vi "Meas Process Record.vi"(5 "result string label":string="str res", 7 "session":T11={"adc"={"niScope"={"channel cfg"=[], "sessions"=[], "multi cards"=FALSE, "channels"=0, "type"=enum."n/a", "memory [B/chn]"=0, "ext. clock [Hz]"=0.0, "samples count"=0, "use streaming"=FALSE, "proc setup"={"packet size [smpl]"=0, "current timeout [s]"=0.0, "blk2blk timeout [s]"=0.0, "event time"=timestamp(0 s since 1904-01-01), "temp sampl T [s]"=0.0, "data queue"=refnum, "stop notifier"=refnum, "proc ref"=refnum}, "sample width [B]"=0, "ranges [V]"=[], "trigger setup"={"coupling"=1, "level [V]"=0.0, "slope"=0, "mode"=enum."Immediate", "pre-trigger [%]"=0.0}, "fs [Hz]"=0.0, "bitres [bit]"=0, "clock source"=enum."VAL_NO_SOURCE"}, "3458A"={"channels"=[], "sync unit"={"VISA"="", "type"=enum."Picotest U6200A"}, "awg unit"={"type"=enum."Agilent 331xxA to 332xxA", "VISA"="", "enable 10MHz ref"=FALSE, "cmi ckd2"={"VISA"="", "clock source"=enum."Auto", "manual ref clk"=FALSE, "ref clock [Hz]"=0.0, "div mode"=enum."Set divisor directly"}, "cmi sync v3"={"VISA"="", "baud rate [bd/s]"=115200, "source"=enum."Auto", "hv range"=enum."1kV", "fsrc is fixed"=FALSE, "fsrc [Hz]"=10000000.0, "freq integ [s]"=1.0, "freq filter"=5, "trig level"=enum."TTL 5V", "chn1 mode"=enum."Source divider", "chn1 level"=enum."Positive 5V", "chn2 mode"=enum."Source divider", "chn2 level"=enum."Positive 5V", "chn2 div"=1, "chn3 mode"=enum."Chn 1 Active", "chn3 level"=enum."Positive 5V", "chn1 div entry"=enum."Calculate nearest divisor from measured fx", "chn1 dev limit [%]"=1.0, "chn1 check dev"=FALSE}, "trigger"={"source"=enum."Immediate", "slope"=enum."POS", "coupling"=enum."DC", "level [V]"=0.0, "hysteresis [V]"=0.0, "pre-trigger [%]"=0.0}, "HMF2500 cfg"={"Baud Rate"=9600, "Parity"=0, "Data Bits"=8, "Flow Control"=4}}, "sync mode"=enum."MASTER-SLAVE, MASTER clocked by TIMER", "streaming mode"=FALSE, "idn mode"=enum."Auto", "sampling mode"=enum."DCV", "sample memory [B]"=0, "proc setup"={"channel id"=0, "packet size [smpl]"=0, "current timeout [s]"=0.0, "blk2blk timeout [s]"=0.0, "event time"=timestamp(0 s since 1904-01-01), "stop notifier"=refnum, "data queues"=[], "proc refs"=[], "bus semaphore"=refnum}, "sample size [B]"=0, "sample count"=0, "aux data"={"channel id"=0, "valid?"=[], "gain [V]"=[], "timestamp [s]"=[], "Ts [s]"=0.0, "abs timestamp"=timestamp(0 s since 1904-01-01), "t [deg C]"=[], "multiplex timestamp [s]"=-1.0, "only multiplex?"=FALSE, "multiplex smpl offset"=0, "overflow?"=FALSE}, "ranges [V]"=[], "aperture [s]"=0.0, "LEVEL trigger"={"edge"=enum."POS", "level [V]"=0.0, "coupling"=enum."DC"}, "trigger mode"=enum."AUTO", "measure temp.?"=FALSE, "disp mesages"=[], "shared bus?"=FALSE, "disable display?"=FALSE, "aper mode"=enum."Manual", "aper rules"=[], "multiplex"={"cycles"=0, "delay [s]"=0.0, "enabled"=FALSE, "overhead [s]"=1.0, "tot smpls"=0, "sub-rec"=0, "overhead [%]"=0.0, "emulated"=FALSE}, "F8588 lpf"=enum."Off", "F8588 pll"=enum."Off", "F8588 couple"=enum."DC, auto", "fs"={"freq mode"=enum."fs or Ts", "fs [Hz]"=0.0, "fref [Hz]"=0.0, "mul"=0.0, "div"=0.0}, "fs mode"=enum."fs or Ts", "init timestamp"=timestamp(0 s since 1904-01-01), "last report timestamp"=timestamp(0 s since 1904-01-01)}, "dsdll"={"dsdll"={"dsdll path"=path "", "dsdll handle"=[], "output devices"=[], "capture devices"=[]}, "channels"=0, "device id"=0, "channel idns"=[], "proc setup"={"packet size [smpl]"=0, "current timeout [s]"=0.0, "blk2blk timeout [s]"=0.0, "event time"=timestamp(0 s since 1904-01-01), "data queue"=refnum, "stop notifier"=refnum, "proc ref"=refnum}, "samples count"=0, "fs [Hz]"=0.0}, "type"=enum."niScope", "channel idn str"=[], "aux instr idn str"=[], "modified?"=FALSE, "simadc"={"channels"=[], "range [V]"=0.0, "Ts step [s]"=0.0, "time [s]"=0.0, "fs [Hz]"=0.0, "count"=0, "smpl offset"=0, "set count"=0, "bit res"=0}, "force rst?"=FALSE, "exit mode"=enum."Immediate reset", "exit dly"=0.0, "exit tmr"=timestamp(0 s since 1904-01-01), "busy?"=FALSE, "accessed?"=FALSE, "multiplex"={"Type"=enum."Dummy", "gen com ssn"={"visa"="", "primary"=enum."None", "secondary"=enum."None", "channels"=[]}, "delay before [s]"=0.0, "delay post [s]"=0.0, "sequence"=[], "enabled"=FALSE, "ref timestamp [s]"=0.0, "idn string"="", "dev niScope"="", "niScope idx"=0, "QPMX ssn"={"visa"="", "switch mode"=enum."Switched by TWM", "sequence"=[], "timing delays"=[], "polarity"=enum."Positive", "ss delay (s)"=2.0, "internal timer (s)"=1.0, "Last loaded sequence file"=path "", "startup delay (s)"=2.0}, "VISA mux ssn"={"VISA"="", "paths"=[], "idn command"="", "serial cfg"={"Baud rate"=9600, "Data bits"=8, "Parity"=0, "Stop bits"=10, "Flow control"=0, "End Mode Read"=enum."None", "End Mode Write"=enum."None", "Term character"=0, "Term enable"=FALSE}}}, "keysight dso"={"VISA"="", "channels"=[], "bw limit [Hz]"=0.0, "resolution"=enum."Basic", "trig noise reject"=enum."Normal", "N"=0, "trigger config"={"trigger source"=enum."Immediate", "trigger slope"=enum."Negative", "level [V]"=0.0, "hysteresis [V]"=0.001, "pre-trig [%]"=50}, "fs [Hz]"=0.0, "timeout stop"=timestamp(0 s since 1904-01-01), "waiting for opc"=FALSE, "fetch offset [smpl]"=0, "abs timestamp"=timestamp(0 s since 1904-01-01), "ranges [V]"=[], "decimation"=1.0, "ext ref"=FALSE, "emulate aperture"=FALSE, "model"=enum."DSO91304"}, "cdaq"={"mclk [Hz]"=12800000.0, "ADC task"="", "mclk reference"="", "fs [Hz]"=50000.0, "queue adc cmd"=refnum, "queue adc data"=refnum, "adc proc ref"=refnum, "channels"=[], "last channels"=[], "timeout"=timestamp(0 s since 1904-01-01), "N"=1000, "mclk mode"=enum."Free running", "ext mclk source"=""}, "ignore overload"=FALSE, "ADS127L21"={"VISA"="", "chn list"=[], "record size"=0, "phys. channels"=0, "adc fifo size"=0, "channels"=[], "ext refclk?"=FALSE, "fs [Hz]"=0.0, "ext refclk [Hz]"=0.0, "meas refclk [Hz]"=0.0, "EXTOUT mode"=enum."ADCCLK", "EXTOUT polarity"=enum."NORM", "EXTOUT divisor"=0}}, "sequence"=[], "sequence setup"={"group setups"=[], "rec count"=0, "range mode"=enum."Keep defaults", "fs mode"=enum."Frequency", "rng even"=0.0, "rng odd"=0.0, "folder"=path "", "name base"="", "meas id"=0, "settle [s]"=0.0, "comment"="", "avg count"=0, "fs-abs-fr fr"=0.0, "fs-abs-fr fs"=0.0, "fs-div fr"=0.0, "fs-div div"=0.0, "fs-mn fr"=0.0, "fs-mn mul"=0.0, "fs-mn div"=0.0, "fs-rat fr"=0.0, "fs-rat rat"=0.0}, "golpi"=refnum, "processing setup"={"mode"=enum."Raw", "call after avgs?"=FALSE, "calculate?"=FALSE, "raw mode"={"command"="", "result mode"=enum."Display console output (only Octave)", "res variable"=""}, "QWTB"={"QWTB path"=path "", "alg filter path"="", "alg ids"=[], "alg parameters"=[], "parsed parameters"=[], "selected alg id"="", "selected unc mode"=enum."None", "qwtb mcc"=100, "qwtb timeout"=90, "qwtb covg"=95.0, "qwtb ofs"=0, "qwtb lim data"=0, "multicore"={"jobs folder"=path "", "cores"=0, "max jobs"=0, "mode"=enum."Singlecore"}, "unc once?"=FALSE, "qwtb tstemp"=enum."Enabled (default)", "octave reset"=FALSE, "exec mode"=enum."Single-core"}}, "corrections"={"transducers"={"channels"=[], "last path"=path "", "root path"=path ""}, "digitizer"={"last path"=path "", "channel paths"=[], "channel idns"=[], "correction name"="", "channel names"=[], "folders to copy"=[], "channel valid"=[], "correction path"=path "", "correction rel path"="", "rel folders to copy"=[], "root path"=path ""}}, "assist cfg"={"P"=0, "Q"=0, "rel shift"=0.0, "ref freq"=0.0, "min fs"=0.0, "max fs tol"=0.0, "min int"=0.0, "max int"=0.0, "max err"=0.0, "max timeout"=0.0}} {"corrections"."transducers"."channels"."Phase index" min=1 step=1; "adc"."ADS127L21"."channels"."Channel" min=1 max=8 step=1; "adc"."ADS127L21"."channels"."Range [Vpk]" items=["±1.65V", "±2V"]; "adc"."cdaq"."last channels"."Channel id" min=0 step=1; "adc"."cdaq"."channels"."Channel id" min=0 step=1; "adc"."keysight dso"."decimation" min=1.0; "adc"."keysight dso"."bw limit [Hz]" format="%#_6p"; "adc"."keysight dso"."channels"."Offset [V]" format="%#_6p"; "adc"."keysight dso"."channels"."Range [Vpk]" min=0.0 format="%#_6p"; "adc"."keysight dso"."channels"."Channel" min=1; "adc"."multiplex"."VISA mux ssn"."serial cfg"."Flow control" items=["None", "XON/XOFF", "CTS/RTS", "XON/XOFF + CTS/RTS", "DTR/DSR", "XON/XOFF + DTR/DSR"]; "adc"."multiplex"."VISA mux ssn"."serial cfg"."Stop bits" items=["1 bit"=10, "1.5 bits"=15, "2 bits"=20]; "adc"."multiplex"."VISA mux ssn"."serial cfg"."Parity" items=["None", "Odd", "Even", "Mark", "Space"]; "adc"."multiplex"."VISA mux ssn"."serial cfg"."Data bits" items=["5 bits"=5, "6 bits"=6, "7 bits"=7, "8 bits"=8]; "adc"."multiplex"."VISA mux ssn"."serial cfg"."Baud rate" items=["150 Bd"=150, "300 Bd"=300, "600 Bd"=600, "1200 Bd"=1200, "2400 Bd"=2400, "4800 Bd"=4800, "9600 Bd"=9600, "19.2 kBd"=19200, "38.4 kBd"=38400, "57.6 kBd"=57600, "115.2 kBd"=115200]; "adc"."multiplex"."QPMX ssn"."startup delay (s)" min=0.0 step=1.0; "adc"."multiplex"."QPMX ssn"."internal timer (s)" min=0.0 step=1.0; "adc"."multiplex"."QPMX ssn"."ss delay (s)" min=0.0 step=1.0; "adc"."multiplex"."QPMX ssn"."timing delays" min=1 max=255 step=1; "adc"."3458A"."awg unit"."HMF2500 cfg"."Flow Control" items=["None", "XON/XOFF", "RTS/CTS", "XON/XOFF & RTS/CTS", "DTR/DSR", "XON/XOFF & DTR/DSR"]; "adc"."3458A"."awg unit"."HMF2500 cfg"."Data Bits" items=["7"=7, "8"=8]; "adc"."3458A"."awg unit"."HMF2500 cfg"."Parity" items=["None", "Odd", "Even", "Mark", "Space"]; "adc"."3458A"."awg unit"."HMF2500 cfg"."Baud Rate" items=["300"=300, "600"=600, "1200"=1200, "2400"=2400, "4800"=4800, "9600"=9600, "19200"=19200]; "adc"."3458A"."awg unit"."cmi sync v3"."chn2 div" min=1 max=100000000 step=1; "adc"."3458A"."awg unit"."cmi sync v3"."fsrc [Hz]" format="%_8p"; "adc"."3458A"."channels"."Range [Vpk]" min=0.0; "adc"."niScope"."trigger setup"."pre-trigger [%]" format="%.2f"; "adc"."niScope"."trigger setup"."level [V]" format="%.2f"; "adc"."niScope"."trigger setup"."coupling" items=["AC"=0, "DC"=1, "HF Reject"=3, "LF Reject"=4, "AC Plus HF Reject"=1001]; "adc"."niScope"."channel cfg"."Range [Vpk]" min=0.0; "adc"."niScope"."channel cfg"."Channel" min=0}, 8 "error in":errorcluster, 10 "group time stamp":timestamp, 11 "sequence item":T2) -> (0 "error out":errorcluster, 2 "new result?":bool)   [LabVIEW 2020]
doc: "Processes record defined by sequence item. It executes code defined in 'sequence setup' passed in the 'session'. It executes the command only if calculation is enabled in the sequence setup. Result from Octave console is printed to the named string using SGUI lib.\nIn QWTB execution mode it either executes alg. directly or in parallel execution mode cretes job file and returns immediately while processing is done by another process(es).\n'group timestamp' is timestamp used to create jobs group for parallel exection mode."
uses:
  Meas Session.ctl
  adc/ADC Session.ctl
  drivers/niScope/niScope Session.ctl
  drivers/niScope/niScope Virtual Channel Config.ctl
  drivers/niScope/niScope Virtual Channel Mode.ctl
  drivers/niScope/niScope Virtual Channel Input Z.ctl
  drivers/niScope/niScope Virtual Channel Coupling.ctl
  drivers/niScope/niScope Type.ctl
  drivers/niScope/niScope Digitizing Process Options.ctl
  drivers/niScope/niScope Data Packet.ctl
  drivers/niScope/niScope Trigger Setup.ctl
  <instrlib>/niScope/Controls/niScope trigger coupling.ctl
  <instrlib>/niScope/Controls/niScope trigger slope.ctl
  drivers/niScope/niScope Reference Clock.ctl
  drivers/DMM/3458A Digitizer Session.ctl
  drivers/DMM/3458A Virtual Channel Config.ctl
  drivers/Counter/Counter Session.ctl
  drivers/Counter/Counter Type.ctl
  drivers/AWG/AWG Session.ctl
  drivers/AWG/AWG Type.ctl
  drivers/AWG/CMI Clock Divider v2/CMI ckd2 Session.ctl
  drivers/AWG/CMI Clock Divider v2/CMI ckd2 Source Mode.ctl
  drivers/AWG/CMI Clock Divider v2/CMI ckd2 Divisor Mode.ctl
  drivers/AWG/CMI Sync V3/CMI Sync V3 session.ctl
  drivers/AWG/CMI Sync V3/Configure/CMI Sync V3 Reference Clock Source.ctl
  drivers/AWG/CMI Sync V3/Configure/CMI Sync V3 HV input Range.ctl
  drivers/AWG/CMI Sync V3/Configure/CMI Sync V3 Trigger Input Level.ctl
  drivers/AWG/CMI Sync V3/Configure/CMI Sync V3 Channel 1 Mode.ctl
  drivers/AWG/CMI Sync V3/Configure/CMI Sync V3 Channel Output Levels.ctl
  drivers/AWG/CMI Sync V3/Configure/CMI Sync V3 Channel 2 Mode.ctl
  drivers/AWG/CMI Sync V3/Configure/CMI Sync V3 Channel 3 Mode.ctl
  drivers/AWG/CMI Sync V3/Configure/CMI Sync V3 Channel 1 Divisor Entry Mode.ctl
  adc/ADC Trig Config.ctl
  adc/ADC Trig Mode Source.ctl
  adc/ADC Trig Slope.ctl
  adc/ADC Trig Coupling.ctl
  drivers/AWG/RaS HMF2500/HMF2500 Config.ctl
  drivers/DMM/3458A Sync Mode.ctl
  drivers/DMM/3458A Idn Mode.ctl
  drivers/DMM/3458A Digitizing Low Levels/Configure/Sampling Mode.ctl
  drivers/DMM/3458A Digitizing Process Options.ctl
  drivers/DMM/3458A Data Packet.ctl
  drivers/DMM/3458A Aux Record Data.ctl
  drivers/DMM/3458A Digitizing Low Levels/Configure/Level Setup.ctl
  drivers/DMM/3458A Digitizing Low Levels/Configure/First Sample Trigger.ctl
  drivers/DMM/3458A Aperture Selection Mode.ctl
  drivers/DMM/3458A Multiplexing Config.ctl
  drivers/Fluke 8588A/F8588A Low Pass Filter.ctl
  drivers/Fluke 8588A/F8588A Phase Lock.ctl
  drivers/Fluke 8588A/F8588A Coupling.ctl
  drivers/DMM/3458A Sampling Rate.ctl
  drivers/AWG/AWG Clock Setup Mode.ctl
  drivers/DMM/3458A Sample Rate Mode.ctl
  drivers/dsdll/DSDLL Session.ctl
  drivers/dsdll/dsdll/dsdll_instance.ctl
  drivers/dsdll/dsdll/dsdll_device_record.ctl
  drivers/dsdll/DSDLL Process Config.ctl
  drivers/dsdll/DSDLL Data Packet.ctl
  adc/ADC Type.ctl
  drivers/simulated_adc/SimAdc Config.ctl
  drivers/simulated_adc/SimAdc Channel Cfg.ctl
  adc/ADC On Close Action.ctl
  adc/Multiplexer/MPX Session.ctl
  adc/Multiplexer/MPX Type.ctl
  drivers/Multiplexers/Generic COM/GCOMM Session.ctl
  drivers/Multiplexers/Generic COM/GCOMM Signal.ctl
  drivers/Multiplexers/Generic COM/GCOMM Virtual Channel.ctl
  drivers/Multiplexers/Generic COM/GCOMM Logic State.ctl
  drivers/Multiplexers/Generic COM/QPMX Session.ctl
  drivers/Multiplexers/QPMX/QPMX switch mode.ctl
  drivers/Multiplexers/QPMX/QPMX polarity.ctl
  drivers/Multiplexers/Generic VISA commands/GVISA Mux Session.ctl
  drivers/Multiplexers/Generic VISA commands/GVISA Mux Path Entry.ctl
  drivers/Multiplexers/Generic VISA commands/met_serial_setup.ctl
  drivers/Agilent DSO 90000/Virtual Digitizer/KeDSO session.ctl
  drivers/Agilent DSO 90000/Virtual Digitizer/KeDSO Virtual Channel.ctl
  drivers/Agilent DSO 90000/Virtual Digitizer/KeDSO High Resolution Mode.ctl
  drivers/Agilent DSO 90000/Virtual Digitizer/KeDSO Trigger Setup.ctl
  drivers/Agilent DSO 90000/Virtual Digitizer/KeDSO Trigger Source.ctl
  drivers/Agilent DSO 90000/Public/Utility/DSO type.ctl
  drivers/cdaq/cDAQ Session.ctl
  drivers/cdaq/low_level_old/cdaq_anal_adc_command.ctl
  drivers/cdaq/low_level_old/cdaq_anal_adc_data.ctl
  drivers/cdaq/cDAQ Virtual Channel.ctl
  drivers/cdaq/cDAQ Master Clock Mode.ctl
  drivers/CMI_ADS127L21/CMI ADS127L21 - Session.ctl
  drivers/CMI_ADS127L21/CMI ADS127L21 - Record Channel.ctl
  drivers/CMI_ADS127L21/CMI ADS127L21 - Input Range.ctl
  drivers/CMI_ADS127L21/CMI ADS127L21 - Input Mode.ctl
  drivers/CMI_ADS127L21/CMI ADS127L21 - Input Impedance.ctl
  drivers/CMI_ADS127L21/CMI ADS127L21 - EXTOUT Mode.ctl
  drivers/CMI_ADS127L21/CMI ADS127L21 - EXTOUT Polarity.ctl
  Meas Sequence Item.ctl
  Meas Sampling Configuration.ctl
  QWTB/Meas Proc QWTB Algorithm Parameter Data.ctl
  Meas Sequence Configuration.ctl
  Meas Range Mode.ctl
  Meas Sampling Rate Mode.ctl
  octave/golpi/mpc/golpi_session_ref.ctl
  octave/golpi/mpc/golpi_session.ctl
  octave/golpi/GOLPI reference Type Def.ctl
  octave/golpi/Pipe Handle.ctl
  Meas Process Config.ctl
  Meas Process Mode.ctl
  Meas Process Raw Config.ctl
  Meas Process Raw Result Mode.ctl
  QWTB/Meas Proc QWTB Setup.ctl
  QWTB/Meas Proc QWTB Uncertainty Mode.ctl
  QWTB/Meas Proc QWTB Multicore Setup.ctl
  QWTB/Meas Proc QWTB Multicore Type.ctl
  Meas Process Time Stamp Mode.ctl
  QWTB/Meas Proc QWTB Exec Mode.ctl
  Corrections/Corr Setup.ctl
  Corrections/Corr Tranducer Item.ctl
  Corrections/Corr Digitizers.ctl
  Assist/Assist Panel Setup.ctl
  varilib/SGUI Assign Multiple Strings With Tags By Label.vi
  octave/golpi/Get String.vi
  varilib/varilib.lvlib
  octave/golpi/mpc/GOLPI Multi Process.lvlib
  octave/golpi/GOLPI library.lvlib
  drivers/niScope/niScope Virtual Digitizer.lvlib
  drivers/DMM/3458A Virtual Digitizer.lvlib
  drivers/Counter/Counter.lvlib
  drivers/AWG/AWG.lvlib
  drivers/DMM/3458A Digitizing Low Levels/3458A Digitizing Low Levels.lvlib
  drivers/dsdll/DSDLL Virtual Digitizer.lvlib
  drivers/dsdll/dsdll/dsdll.lvlib
  octave/golpi/LV Process library.lvlib
  drivers/AWG/CMI Sync V3/CMI Sync Unit V3.lvlib
  drivers/Agilent DSO 90000/Agilent 90000 Series.lvlib
panel:
  in  "mode":T1
  # "ADC:"
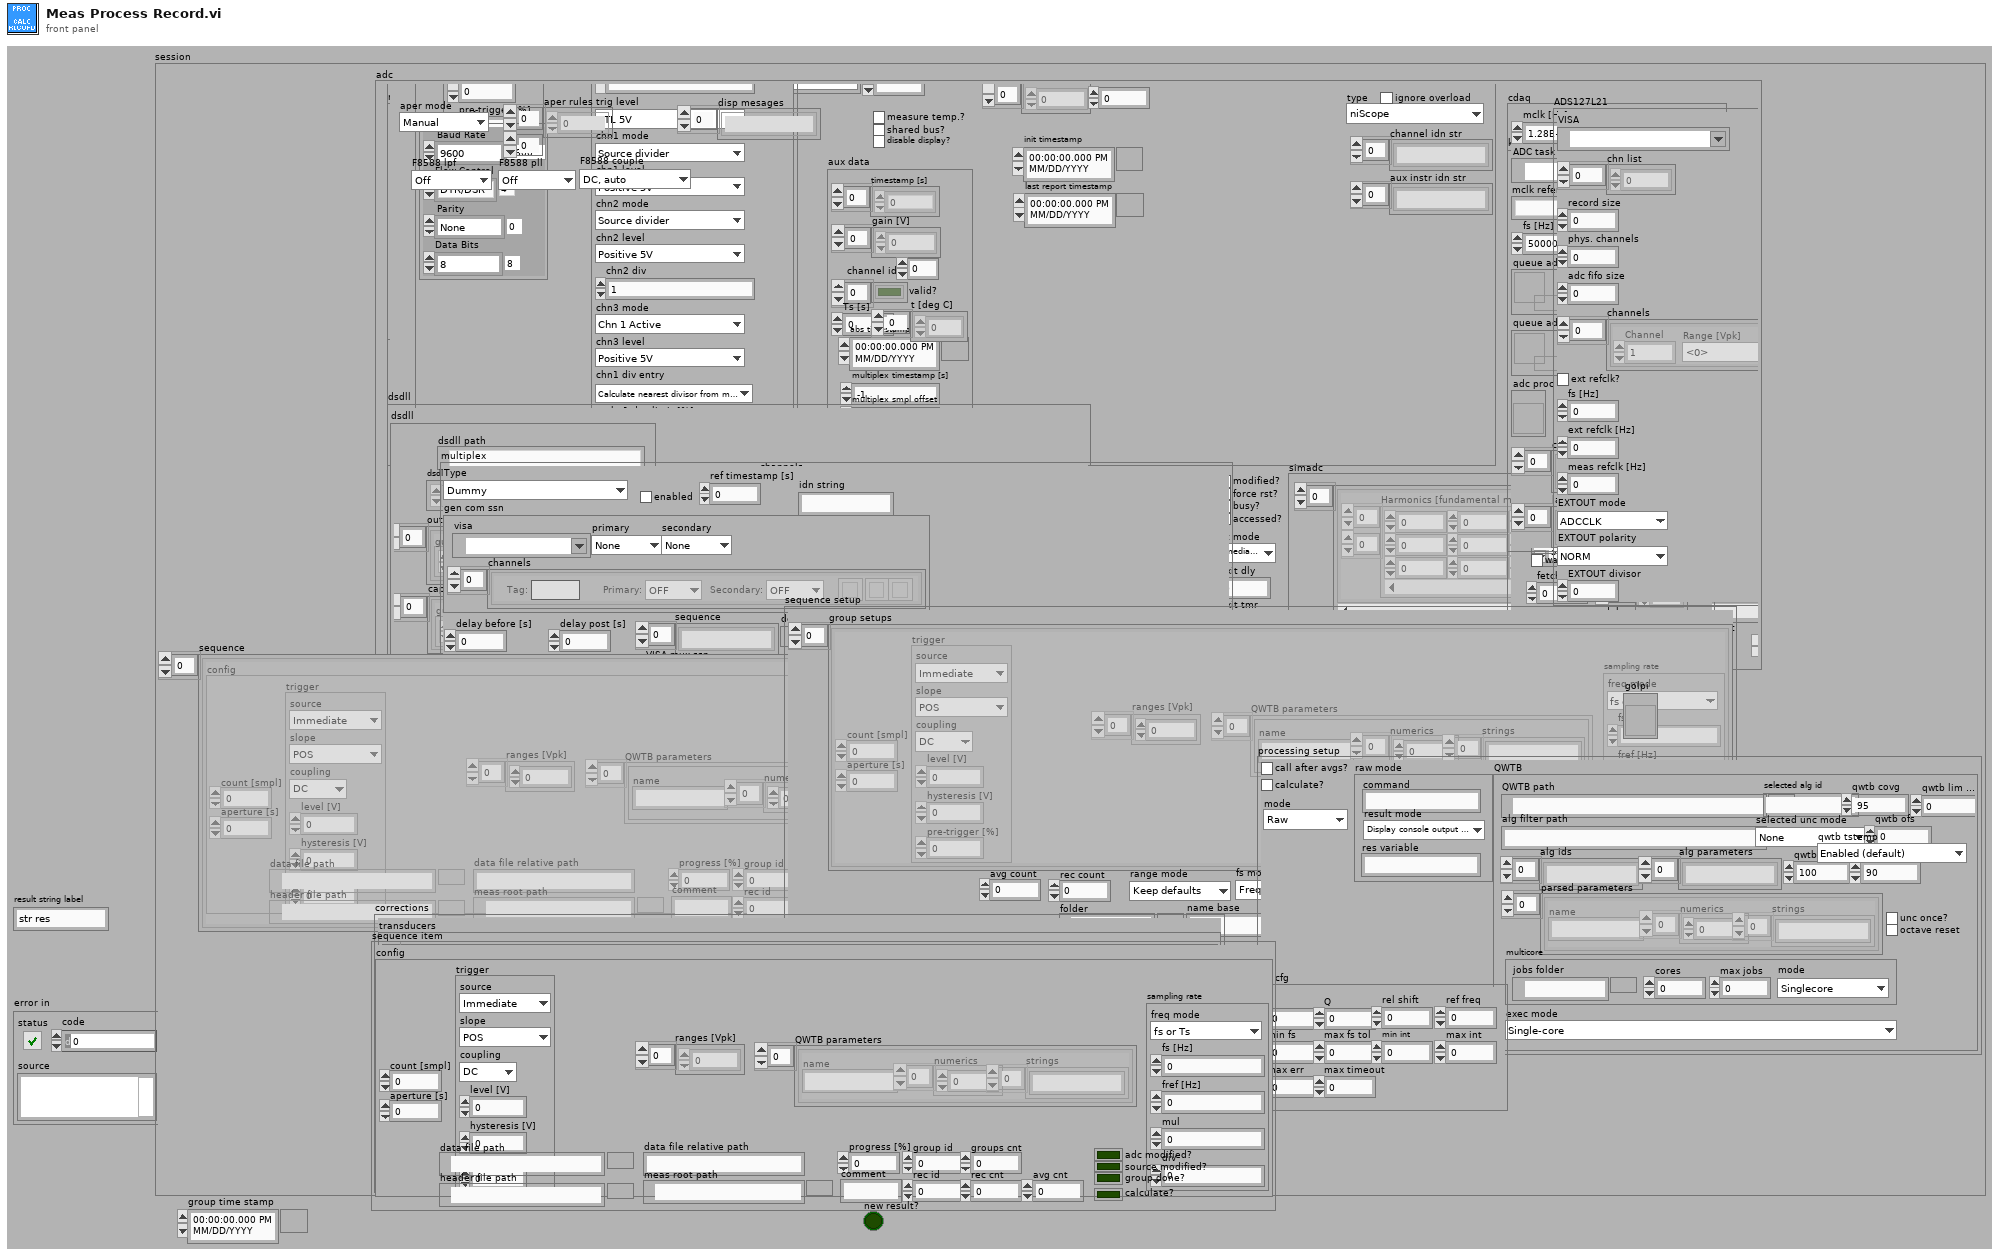
[diagram p1: front panel]
types:
  T1 = typedef "Meas Proc QWTB Multicore Type.ctl" = enum16{"Singlecore", "Multicore", "Multistation"}
  T2 = typedef "Meas Sequence Item.ctl" = cluster{"config":T3, "data file path":path, "header file path":path, "group id":i32, "rec id":i32, "group done?":bool, "adc modified?":bool, "source modified?":bool, "progress [%]":dbl, "groups cnt":i32, "rec cnt":i32, "data file relative path":string, "meas root path":path, "calculate?":bool, "comment":string, "avg cnt":i32}
  T3 = typedef "Meas Sampling Configuration.ctl" = cluster{"count [smpl]":i64, "aperture [s]":dbl, "trigger":T4, "ranges [Vpk]":dbl[], "QWTB parameters":T8[], "sampling rate":T9}
  T4 = typedef "ADC Trig Config.ctl" = cluster{"source":T5, "slope":T6, "coupling":T7, "level [V]":dbl, "hysteresis [V]":dbl, "pre-trigger [%]":dbl}
  T5 = typedef "ADC Trig Mode Source.ctl" = enum16{"Immediate", "External", "Level"}
  T6 = typedef "ADC Trig Slope.ctl" = enum16{"POS", "NEG"}
  T7 = typedef "ADC Trig Coupling.ctl" = enum16{"DC", "AC"}
  T8 = typedef "Meas Proc QWTB Algorithm Parameter Data.ctl" = cluster{"name":string, "numerics":dbl[], "strings":string[]}
  T9 = typedef "3458A Virtual Digitizer.lvlib/3458A Sampling Rate.ctl" = cluster{"freq mode":T10, "fs [Hz]":dbl, "fref [Hz]":dbl, "mul":dbl, "div":dbl}
  T10 = typedef "AWG.lvlib/AWG Clock Setup Mode.ctl" = enum16{"fs or Ts", "fs or Ts with fref", "fref/N", "fref*M/N", "fref*Ratio"}
  T11 = typedef "Meas Session.ctl" = cluster{"adc":T12, "sequence":T2[], "sequence setup":T93, "golpi":T96, "processing setup":T97, "corrections":T106, "assist cfg":T109}
  T12 = typedef "ADC Session.ctl" = cluster{"niScope":T13, "3458A":T24, "dsdll":T57, "type":T61, "channel idn str":string[], "aux instr idn str":string[], "modified?":bool, "simadc":T62, "force rst?":bool, "exit mode":T64, "exit dly":dbl, "exit tmr":timestamp, "busy?":bool, "accessed?":bool, "multiplex":T65, "keysight dso":T77, "cdaq":T83, "ignore overload":bool, "ADS127L21":T86}
  T13 = typedef "niScope Virtual Digitizer.lvlib/niScope Session.ctl" = cluster{"channel cfg":T14[], "sessions":refnum<k20>[], "multi cards":bool, "channels":i32, "type":T18, "memory [B/chn]":i32, "ext. clock [Hz]":dbl, "samples count":i64, "use streaming":bool, "proc setup":T19, "sample width [B]":i32, "ranges [V]":dbl[], "trigger setup":T20, "fs [Hz]":dbl, "bitres [bit]":i32, "clock source":T23}
  T14 = typedef "niScope Virtual Digitizer.lvlib/niScope Virtual Channel Config.ctl" = cluster{"Address":refnum<k15>, "Channel":i32, "Mode":T15, "Input Z":T16, "Coupling":T17, "Range [Vpk]":dbl, "btn clr":bool, "btn up":bool, "btn down":bool}
  T15 = typedef "niScope Virtual Digitizer.lvlib/niScope Virtual Channel Mode.ctl" = enum16{"Single ended", "Unbal. differential", "Differential"}
  T16 = typedef "niScope Virtual Digitizer.lvlib/niScope Virtual Channel Input Z.ctl" = enum16{"1 MOhm", "50 Ohm"}
  T17 = typedef "niScope Virtual Digitizer.lvlib/niScope Virtual Channel Coupling.ctl" = enum16{"AC", "DC", "GND"}
  T18 = typedef "niScope Virtual Digitizer.lvlib/niScope Type.ctl" = enum16{"n/a", "5922"}
  T19 = typedef "niScope Virtual Digitizer.lvlib/niScope Digitizing Process Options.ctl" = cluster{"packet size [smpl]":i64, "current timeout [s]":dbl, "blk2blk timeout [s]":dbl, "event time":timestamp, "temp sampl T [s]":dbl, "data queue":refnum<queue>, "stop notifier":refnum<notifier>, "proc ref":refnum<vi>}
  T20 = typedef "niScope Virtual Digitizer.lvlib/niScope Trigger Setup.ctl" = cluster{"coupling":T21, "level [V]":dbl, "slope":T22, "mode":enum16{"Immediate", "External", "Level"}, "pre-trigger [%]":dbl}
  T21 = typedef "niScope trigger coupling.ctl" = u16
  T22 = typedef "niScope trigger slope.ctl" = i32
  T23 = typedef "niScope Virtual Digitizer.lvlib/niScope Reference Clock.ctl" = enum16{"VAL_NO_SOURCE", "VAL_CLK_IN", "VAL_PXI_CLOCK", "VAL_EXTERNAL"}
  T24 = typedef "3458A Virtual Digitizer.lvlib/3458A Digitizer Session.ctl" = cluster{"channels":T25[], "sync unit":T26, "awg unit":T28, "sync mode":T43, "streaming mode":bool, "idn mode":T44, "sampling mode":T45, "sample memory [B]":i32, "proc setup":T46, "sample size [B]":i32, "sample count":i32, "aux data":T48, "ranges [V]":dbl[], "aperture [s]":dbl, "LEVEL trigger":T49, "trigger mode":T50, "measure temp.?":bool, "disp mesages":string[], "shared bus?":bool, "disable display?":bool, "aper mode":T51, "aper rules":dbl[][], "multiplex":T52, "F8588 lpf":T53, "F8588 pll":T54, "F8588 couple":T55, "fs":T9, "fs mode":T56, "init timestamp":timestamp, "last report timestamp":timestamp}
  T25 = typedef "3458A Virtual Digitizer.lvlib/3458A Virtual Channel Config.ctl" = cluster{"VISA":refnum<visa-resource-name>, "Range [Vpk]":dbl, "btn clr":bool, "btn up":bool, "btn down":bool, "F8588":bool, "F8588 guard":bool}
  T26 = typedef "Counter.lvlib/Counter Session.ctl" = cluster{"VISA":refnum<visa-resource-name>, "type":T27}
  T27 = typedef "Counter.lvlib/Counter Type.ctl" = enum16{"Picotest U6200A", "dummy"}
  T28 = typedef "AWG.lvlib/AWG Session.ctl" = cluster{"type":T29, "VISA":refnum<visa-resource-name>, "enable 10MHz ref":bool, "cmi ckd2":T30, "cmi sync v3":T33, "trigger":T4, "HMF2500 cfg":T42}
  T29 = typedef "AWG.lvlib/AWG Type.ctl" = enum16{"Agilent 331xxA to 332xxA", "Agilent 335xxA to 336xxA", "Tektronix AFG3101C", "R&S HMF25xx", "CMI Clock Divider v2", "CMI Sync Unit V3", "dummy"}
  T30 = typedef "AWG.lvlib/CMI ckd2 Session.ctl" = cluster{"VISA":refnum<visa-resource-name>, "clock source":T31, "manual ref clk":bool, "ref clock [Hz]":dbl, "div mode":T32}
  T31 = typedef "AWG.lvlib/CMI ckd2 Source Mode.ctl" = enum16{"Auto", "LF clock", "HF clock", "Internal"}
  T32 = typedef "AWG.lvlib/CMI ckd2 Divisor Mode.ctl" = enum16{"Set divisor directly", "Set divisor by frequency"}
  T33 = typedef "AWG.lvlib/CMI Sync Unit V3.lvlib/CMI Sync V3 session.ctl" = cluster{"VISA":refnum<visa-resource-name>, "baud rate [bd/s]":i32, "source":T34, "hv range":T35, "fsrc is fixed":bool, "fsrc [Hz]":dbl, "freq integ [s]":dbl, "freq filter":i32, "trig level":T36, "chn1 mode":T37, "chn1 level":T38, "chn2 mode":T39, "chn2 level":T38, "chn2 div":i32, "chn3 mode":T40, "chn3 level":T38, "chn1 div entry":T41, "chn1 dev limit [%]":dbl, "chn1 check dev":bool}
  T34 = typedef "AWG.lvlib/CMI Sync Unit V3.lvlib/CMI Sync V3 Reference Clock Source.ctl" = enum16{"Auto", "Internal", "Logic", "Sine", "HV"}
  T35 = typedef "AWG.lvlib/CMI Sync Unit V3.lvlib/CMI Sync V3 HV input Range.ctl" = enum16{"10V", "60V", "250V", "1kV"}
  T36 = typedef "AWG.lvlib/CMI Sync Unit V3.lvlib/CMI Sync V3 Trigger Input Level.ctl" = enum16{"LVCMOS 3V3", "TTL 5V"}
  T37 = typedef "AWG.lvlib/CMI Sync Unit V3.lvlib/CMI Sync V3 Channel 1 Mode.ctl" = enum16{"Source divider", "DDS absolute", "DDS ratio", "DDS ratio M/N"}
  T38 = typedef "AWG.lvlib/CMI Sync Unit V3.lvlib/CMI Sync V3 Channel Output Levels.ctl" = enum16{"Positive 3V3", "Negative 3V3", "Positive 5V", "Negative 5V"}
  T39 = typedef "AWG.lvlib/CMI Sync Unit V3.lvlib/CMI Sync V3 Channel 2 Mode.ctl" = enum16{"Source divider", "Chn 1 divide"}
  T40 = typedef "AWG.lvlib/CMI Sync Unit V3.lvlib/CMI Sync V3 Channel 3 Mode.ctl" = enum16{"Chn 1 Active", "Chn 2 Active", "Chn 1 Trigger", "Chn 2 Trigger", "Gate", "PPS", "10MHz"}
  T41 = typedef "AWG.lvlib/CMI Sync Unit V3.lvlib/CMI Sync V3 Channel 1 Divisor Entry Mode.ctl" = enum16{"Set divisor directly", "Calculate nearest divisor from measured fx"}
  T42 = typedef "AWG.lvlib/HMF2500 Config.ctl" = cluster{"Baud Rate":u32, "Parity":u16, "Data Bits":u16, "Flow Control":u16}
  T43 = typedef "3458A Virtual Digitizer.lvlib/3458A Sync Mode.ctl" = enum16{"MASTER-SLAVE, MASTER clocked by TIMER", "MASTER-SLAVE, MASTER clocked by AWG", "ALL clocked by AWG", "MASTER-SLAVE, ALL clocked by TIMER", "ALL clocked by AWG with DFLL"}
  T44 = typedef "3458A Virtual Digitizer.lvlib/3458A Idn Mode.ctl" = enum16{"Auto", "Sequential (chn A, chn B, ...)", "From calibration string"}
  T45 = typedef "3458A Virtual Digitizer.lvlib/3458A Digitizing Low Levels.lvlib/Sampling Mode.ctl" = enum16{"DCV", "DSDC", "DSAC"}
  T46 = typedef "3458A Virtual Digitizer.lvlib/3458A Digitizing Process Options.ctl" = cluster{"channel id":i32, "packet size [smpl]":i32, "current timeout [s]":dbl, "blk2blk timeout [s]":dbl, "event time":timestamp, "stop notifier":refnum<notifier>, "data queues":refnum<queue>[], "proc refs":refnum<vi>[], "bus semaphore":T47}
  T47 = typedef "Semaphore RefNum" = refnum<k1>
  T48 = typedef "3458A Virtual Digitizer.lvlib/3458A Aux Record Data.ctl" = cluster{"channel id":i32, "valid?":bool[], "gain [V]":dbl[], "timestamp [s]":dbl[], "Ts [s]":dbl, "abs timestamp":timestamp, "t [deg C]":dbl[], "multiplex timestamp [s]":dbl, "only multiplex?":bool, "multiplex smpl offset":i64, "overflow?":bool}
  T49 = typedef "3458A Virtual Digitizer.lvlib/3458A Digitizing Low Levels.lvlib/Level Setup.ctl" = cluster{"edge":enum16{"POS", "NEG"}, "level [V]":dbl, "coupling":enum16{"DC", "AC"}}
  T50 = typedef "3458A Virtual Digitizer.lvlib/3458A Digitizing Low Levels.lvlib/First Sample Trigger.ctl" = enum16{"AUTO", "EXT", "SYN", "SGL", "HOLD", "LEVEL"}
  T51 = typedef "3458A Virtual Digitizer.lvlib/3458A Aperture Selection Mode.ctl" = enum16{"Manual", "Maximum", "Table"}
  T52 = typedef "3458A Virtual Digitizer.lvlib/3458A Multiplexing Config.ctl" = cluster{"cycles":i32, "delay [s]":dbl, "enabled":bool, "overhead [s]":dbl, "tot smpls":i64, "sub-rec":i32, "overhead [%]":dbl, "emulated":bool}
  T53 = typedef "F8588A Low Pass Filter.ctl" = enum16{"Off", "100 kHz", "3 MHz"}
  T54 = typedef "F8588A Phase Lock.ctl" = enum16{"Off", "1 MHz", "10 MHz"}
  T55 = typedef "F8588A Coupling.ctl" = enum16{"AC, 1 MOhm", "AC, 10 MOhm", "DC, 1 MOhm", "DC, 10 MOhm", "DC, auto"}
  T56 = typedef "3458A Sample Rate Mode.ctl" = enum16{"fs or Ts", "fs*M/N"}
  T57 = typedef "DSDLL Virtual Digitizer.lvlib/DSDLL Session.ctl" = cluster{"dsdll":T58, "channels":i32, "device id":i32, "channel idns":string[], "proc setup":T60, "samples count":i32, "fs [Hz]":dbl}
  T58 = typedef "dsdll.lvlib/dsdll_instance.ctl" = cluster{"dsdll path":path, "dsdll handle":u8[], "output devices":T59[], "capture devices":T59[]}
  T59 = typedef "dsdll.lvlib/dsdll_device_record.ctl" = cluster{"guid":u8[], "name":string}
  T60 = typedef "DSDLL Virtual Digitizer.lvlib/DSDLL Process Config.ctl" = cluster{"packet size [smpl]":i32, "current timeout [s]":dbl, "blk2blk timeout [s]":dbl, "event time":timestamp, "data queue":refnum<queue>, "stop notifier":refnum<notifier>, "proc ref":refnum<vi>}
  T61 = typedef "ADC Type.ctl" = enum16{"niScope", "3458A", "DirectSound DLL", "Keysight DSO", "cDAQ ADC", "CMI ADS127L21", "dummy"}
  T62 = typedef "SimAdc Config.ctl" = cluster{"channels":T63[], "range [V]":dbl, "Ts step [s]":dbl, "time [s]":dbl, "fs [Hz]":dbl, "count":i64, "smpl offset":i64, "set count":i64, "bit res":i32}
  T63 = typedef "SimAdc Channel Cfg.ctl" = cluster{"harmonics":dbl[][], "btn clear":bool, "noise":dbl, "fundamental [Hz]":dbl}
  T64 = typedef "ADC On Close Action.ctl" = enum16{"Immediate reset", "Delayed reset"}
  T65 = typedef "MPX Session.ctl" = cluster{"Type":T66, "gen com ssn":T67, "delay before [s]":dbl, "delay post [s]":dbl, "sequence":string[], "enabled":bool, "ref timestamp [s]":dbl, "idn string":string, "dev niScope":refnum<k15>, "niScope idx":i32, "QPMX ssn":T71, "VISA mux ssn":T74}
  T66 = typedef "MPX Type.ctl" = enum16{"Dummy", "Generic - COM port", "Generic - niScope PFI", "Generic - VISA commands", "QPMX"}
  T67 = typedef "GCOMM Session.ctl" = cluster{"visa":refnum<visa-resource-name>, "primary":T68, "secondary":T68, "channels":T69[]}
  T68 = typedef "GCOMM Signal.ctl" = enum16{"None", "DTR", "RTS"}
  T69 = typedef "GCOMM Virtual Channel.ctl" = cluster{"Primary:":T70, "Secondary:":T70, "btn clr":bool, "btn up":bool, "btn down":bool, "Tag:":string}
  T70 = typedef "GCOMM Logic State.ctl" = enum16{"OFF", "ON"}
  T71 = typedef "QPMX Session.ctl" = cluster{"visa":refnum<visa-resource-name>, "switch mode":T72, "sequence":bool[][], "timing delays":u32[], "polarity":T73, "ss delay (s)":dbl, "internal timer (s)":dbl, "Last loaded sequence file":path, "startup delay (s)":dbl}
  T72 = typedef "QPMX switch mode.ctl" = enum16{"Switched by TWM", "Switched by external clock", "Switched by internal clock"}
  T73 = typedef "QPMX polarity.ctl" = enum16{"Positive", "Negative"}
  T74 = typedef "GVISA Mux Session.ctl" = cluster{"VISA":refnum<visa-resource-name>, "paths":T75[], "idn command":string, "serial cfg":T76}
  T75 = typedef "GVISA Mux Path Entry.ctl" = cluster{"Tag:":string, "Command:":string, "btn clr":bool, "btn up":bool, "btn down":bool}
  T76 = typedef "met_serial_setup.ctl" = cluster{"Baud rate":i32, "Data bits":i32, "Parity":i32, "Stop bits":i32, "Flow control":i32, "End Mode Read":enum16{"None", "Last Bit", "TermChar"}, "End Mode Write":enum16{"None", "Last Bit", "TermChar"}, "Term character":u8, "Term enable":bool}
  T77 = typedef "KeDSO session.ctl" = cluster{"VISA":refnum<visa-resource-name>, "channels":T78[], "bw limit [Hz]":dbl, "resolution":T79, "trig noise reject":enum16{"Normal", "High Sensitivity"}, "N":i64, "trigger config":T80, "fs [Hz]":dbl, "timeout stop":timestamp, "waiting for opc":bool, "fetch offset [smpl]":i64, "abs timestamp":timestamp, "ranges [V]":dbl[], "decimation":dbl, "ext ref":bool, "emulate aperture":bool, "model":T82}
  T78 = typedef "KeDSO Virtual Channel.ctl" = cluster{"Channel":i32, "Range [Vpk]":dbl, "btn clr":bool, "btn up":bool, "btn down":bool, "Offset [V]":dbl, "Coupling":enum16{"DC", "DC50", "AC", "LFR1"}, "bw limit enab":bool}
  T79 = typedef "KeDSO High Resolution Mode.ctl" = enum16{"Basic", "High-res AUTO", "Min. 9-bits", "Min. 10-bits", "Min. 11-bits", "Min. 12-bits", "Fixed 11-bits", "Fixed 12-bits", "Fixed 13-bits", "Fixed 14-bits", "Fixed 15-bits", "Fixed 16-bits"}
  T80 = typedef "KeDSO Trigger Setup.ctl" = cluster{"trigger source":T81, "trigger slope":enum16{"Negative", "Positive", "Either"}, "level [V]":dbl, "hysteresis [V]":dbl, "pre-trig [%]":i32}
  T81 = typedef "KeDSO Trigger Source.ctl" = enum16{"Immediate", "Level", "AUX"}
  T82 = typedef "Agilent 90000 Series.lvlib/DSO type.ctl" = enum16{"DSO91304", "DSO91204", "DSO90804", "DSO90604", "DSO90404", "DSO90254", "DSA91304", "DSA91204", "DSA90804", "DSA90604", "DSA90404", "DSA90254", "DSO9104", "DSO9254", "DSO9404", "MSO9104", "MSO9254", "MSO9404", "MSO9064", "DSO9064", "DSOX91604", "DSOX92004", "DSOX92504", "DSOX92804", "DSOX93204", "DSO93004", "DSO9024H", "DSO9054H", "DSO9104H", "DSO9204H", "DSOS054A", "DSOS104A", "DSOS204A", "DSOS254A", "DSOS404A", "DSOS604A", "DSOS804A", "MSOS054A", "MSOS104A", "MSOS204A", "MSOS254A", "MSOS404A", "MSOS604A", "MSOS804A", "DSAX96204Q", "DSOX96204Q", "DSAX95004Q", "DSOX95004Q", "DSAX93304Q", "DSOX93304Q", "DSAX92504Q", "DSOX92504Q", "DSAX92004Q", "DSOX92004Q"}
  T83 = typedef "cDAQ Session.ctl" = cluster{"mclk [Hz]":dbl, "ADC task":refnum<k21>, "mclk reference":string, "fs [Hz]":dbl, "queue adc cmd":refnum<queue>, "queue adc data":refnum<queue>, "adc proc ref":refnum<vi>, "channels":T84[], "last channels":T84[], "timeout":timestamp, "N":i32, "mclk mode":T85, "ext mclk source":tag}
  T84 = typedef "cDAQ Virtual Channel.ctl" = cluster{"Device":tag, "Channel id":i32, "btn clr":bool, "btn up":bool, "btn down":bool}
  T85 = typedef "cDAQ Master Clock Mode.ctl" = enum16{"Free running", "Export master clock", "Import master clock"}
  T86 = typedef "CMI ADS127L21 - Session.ctl" = cluster{"VISA":refnum<visa-resource-name>, "chn list":i32[], "record size":i32, "phys. channels":i32, "adc fifo size":i32, "channels":T87[], "ext refclk?":bool, "fs [Hz]":dbl, "ext refclk [Hz]":dbl, "meas refclk [Hz]":dbl, "EXTOUT mode":T91, "EXTOUT polarity":T92, "EXTOUT divisor":i32}
  T87 = typedef "CMI ADS127L21 - Record Channel.ctl" = cluster{"Range [Vpk]":T88, "Channel":i32, "Mode":T89, "Impedance":T90, "btn clr":bool, "btn up":bool, "btn down":bool}
  T88 = typedef "CMI ADS127L21 - Input Range.ctl" = dbl
  T89 = typedef "CMI ADS127L21 - Input Mode.ctl" = enum16{"Normal", "Inverted", "GND"}
  T90 = typedef "CMI ADS127L21 - Input Impedance.ctl" = enum16{"1M", "1k5"}
  T91 = typedef "CMI ADS127L21 - EXTOUT Mode.ctl" = enum16{"ADCCLK", "REFCLK", "SMPLCLK", "FIRST"}
  T92 = typedef "CMI ADS127L21 - EXTOUT Polarity.ctl" = enum16{"NORM", "INV"}
  T93 = typedef "Meas Sequence Configuration.ctl" = cluster{"group setups":T3[], "rec count":i32, "range mode":T94, "fs mode":T95, "rng even":dbl, "rng odd":dbl, "folder":path, "name base":string, "meas id":i32, "settle [s]":dbl, "comment":string, "avg count":i32, "fs-abs-fr fr":dbl, "fs-abs-fr fs":dbl, "fs-div fr":dbl, "fs-div div":dbl, "fs-mn fr":dbl, "fs-mn mul":dbl, "fs-mn div":dbl, "fs-rat fr":dbl, "fs-rat rat":dbl}
  T94 = typedef "Meas Range Mode.ctl" = enum16{"Keep defaults", "Set All channels", "Set Odd and Even channels"}
  T95 = typedef "Meas Sampling Rate Mode.ctl" = enum16{"Frequency", "Period"}
  T96 = typedef "GOLPI Multi Process.lvlib/golpi_session_ref.ctl" = refnum<vi>
  T97 = typedef "Meas Process Config.ctl" = cluster{"mode":T98, "call after avgs?":bool, "calculate?":bool, "raw mode":T99, "QWTB":T101}
  T98 = typedef "Meas Process Mode.ctl" = enum16{"Raw", "QWTB"}
  T99 = typedef "Meas Process Raw Config.ctl" = cluster{"command":string, "result mode":T100, "res variable":string}
  T100 = typedef "Meas Process Raw Result Mode.ctl" = enum16{"Display console output (only Octave)", "Display string variable", "Display result file %respath%"}
  T101 = typedef "Meas Proc QWTB Setup.ctl" = cluster{"QWTB path":path, "alg filter path":string, "alg ids":string[], "alg parameters":string[], "parsed parameters":T8[], "selected alg id":string, "selected unc mode":T102, "qwtb mcc":i32, "qwtb timeout":i32, "qwtb covg":dbl, "qwtb ofs":i64, "qwtb lim data":i64, "multicore":T103, "unc once?":bool, "qwtb tstemp":T104, "octave reset":bool, "exec mode":T105}
  T102 = typedef "Meas Proc QWTB Uncertainty Mode.ctl" = enum16{"None", "GUF", "Monte Carlo"}
  T103 = typedef "Meas Proc QWTB Multicore Setup.ctl" = cluster{"jobs folder":path, "cores":i32, "max jobs":i32, "mode":T1}
  T104 = typedef "Meas Process Time Stamp Mode.ctl" = enum16{"Enabled (default)", "Disabled", "Relative to 1. record"}
  T105 = typedef "Meas Proc QWTB Exec Mode.ctl" = enum16{"Single-core", "Parallel Record Processing"}
  T106 = typedef "Corr Setup.ctl" = cluster{"transducers":cluster{"channels":T107[], "last path":path, "root path":path}, "digitizer":T108}
  T107 = typedef "Corr Tranducer Item.ctl" = cluster{"Path":path, "Ratio:":string, "Name:":string, "btn rem":bool, "btn up":bool, "btn down":bool, "s.n.:":string, "btn open":bool, "ratio o/i":dbl, "chn hi":u16, "chn lo":u16, "Phase index":i32, "btn edit":bool, "mpx chn":u16, "btn vdx1":bool, "btn csx1":bool, "invert":bool}
  T108 = typedef "Corr Digitizers.ctl" = cluster{"last path":path, "channel paths":path[], "channel idns":string[], "correction name":string, "channel names":string[], "folders to copy":path[], "channel valid":bool[], "correction path":path, "correction rel path":string, "rel folders to copy":string[], "root path":path}
  T109 = typedef "Assist Panel Setup.ctl" = cluster{"P":i32, "Q":i32, "rel shift":dbl, "ref freq":dbl, "min fs":dbl, "max fs tol":dbl, "min int":dbl, "max int":dbl, "max err":dbl, "max timeout":dbl}
  T110 = typedef "GOLPI library.lvlib/GOLPI reference Type Def.ctl" = cluster{"pipe handle":T111, "fast read timeout [ms]":u32, "fast read settle time [ms]":u32, "fast read to multiple [ms]":u32, "max elements per input line":u32, "slow read timeout [ms]":u32, "stdin double format specifier":string, "max elements per stdout output column":u32, "console mode bitstream":bool, "bitstream first read timeout [ms]":u32, "bitstream read timeout [ms]":u32, "struct transfer possible":bool, "matlab mode":bool}
  T111 = typedef "LV Process library.lvlib/Pipe Handle.ctl" = cluster{"lv_proc.dll file path":path, "process instance handle":u32[], "debug mode":bool, "debug data":cluster{"time":timestamp, "stdin":bool, "data":string}[]}
  T112 = typedef "GOLPI Multi Process.lvlib/golpi_session.ctl" = cluster{"GOLPI ref":T110, "idn str":string, "octave path":path, "work path":path, "start timeout [ms]":u32, "clr cache":bool, "console":bool, "binary":bool, "semaphore":T47, "initial command":string, "exit command":string, "matlab":bool, "pkg list":string[]}
  T113 = typedef "LVDateTimeRec.ctl" = cluster{"fractional second":dbl, "second":i32, "minute":i32, "hour":i32, "day of month":i32, "month":i32, "year":i32, "day of week":i32, "day of year":i32, "DST":i32}
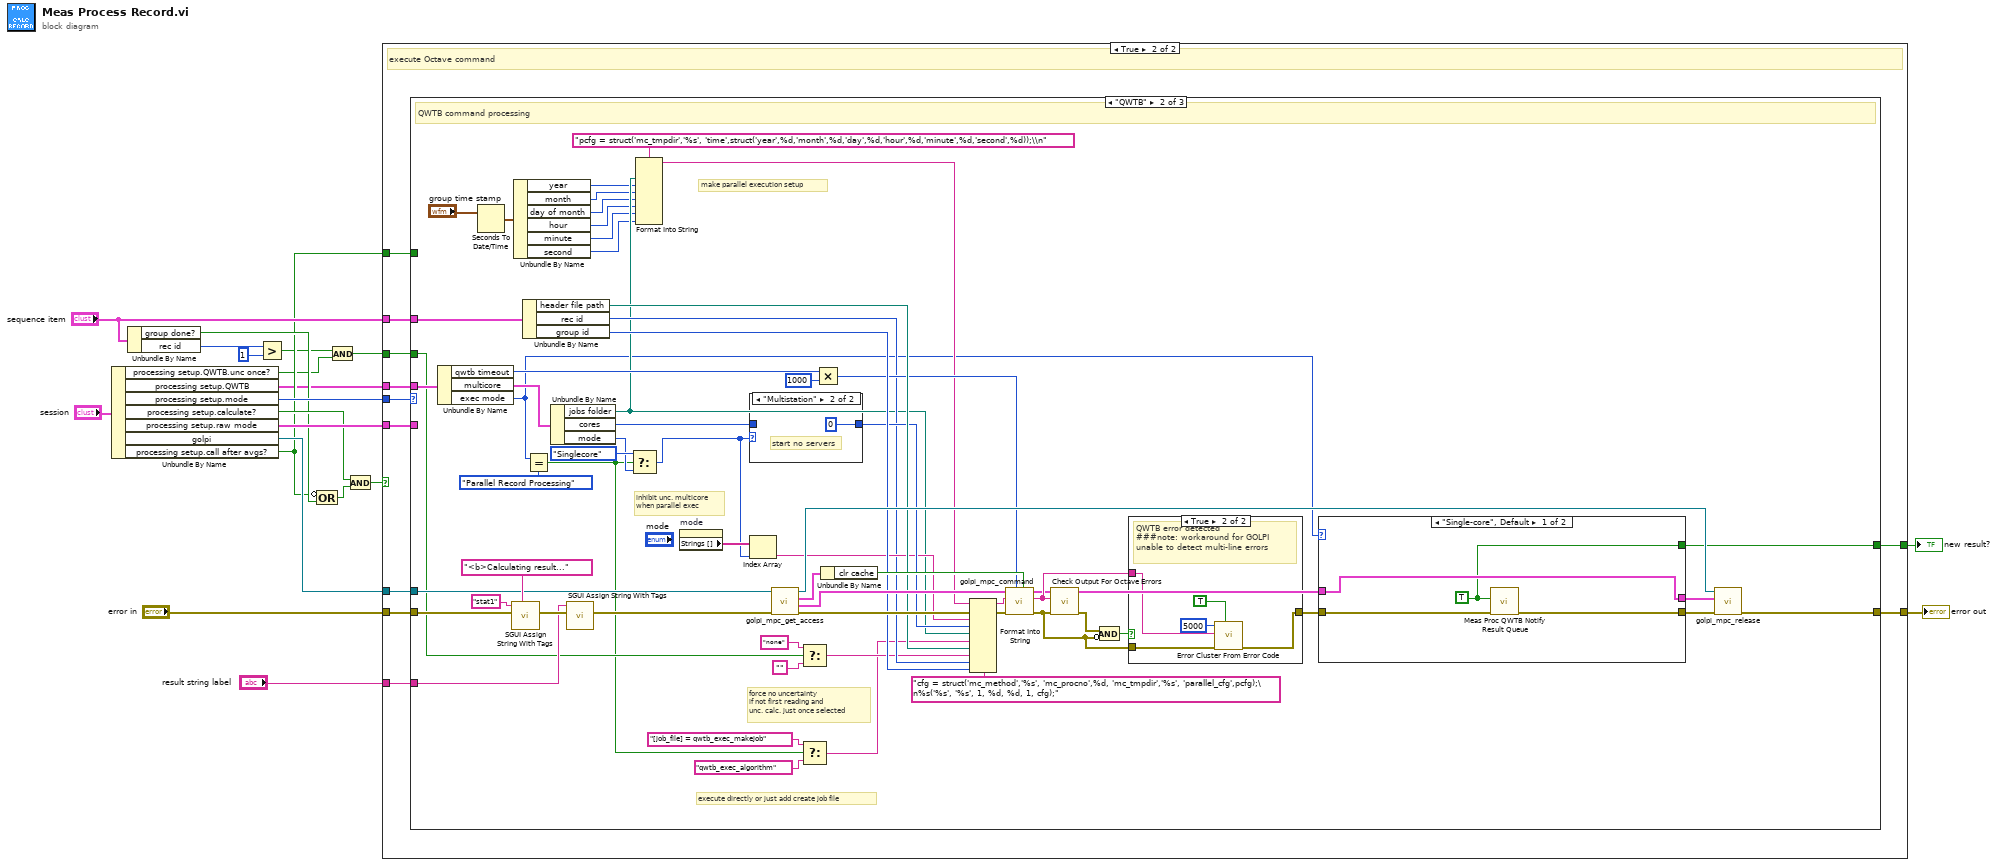
[diagram p0: block diagram]
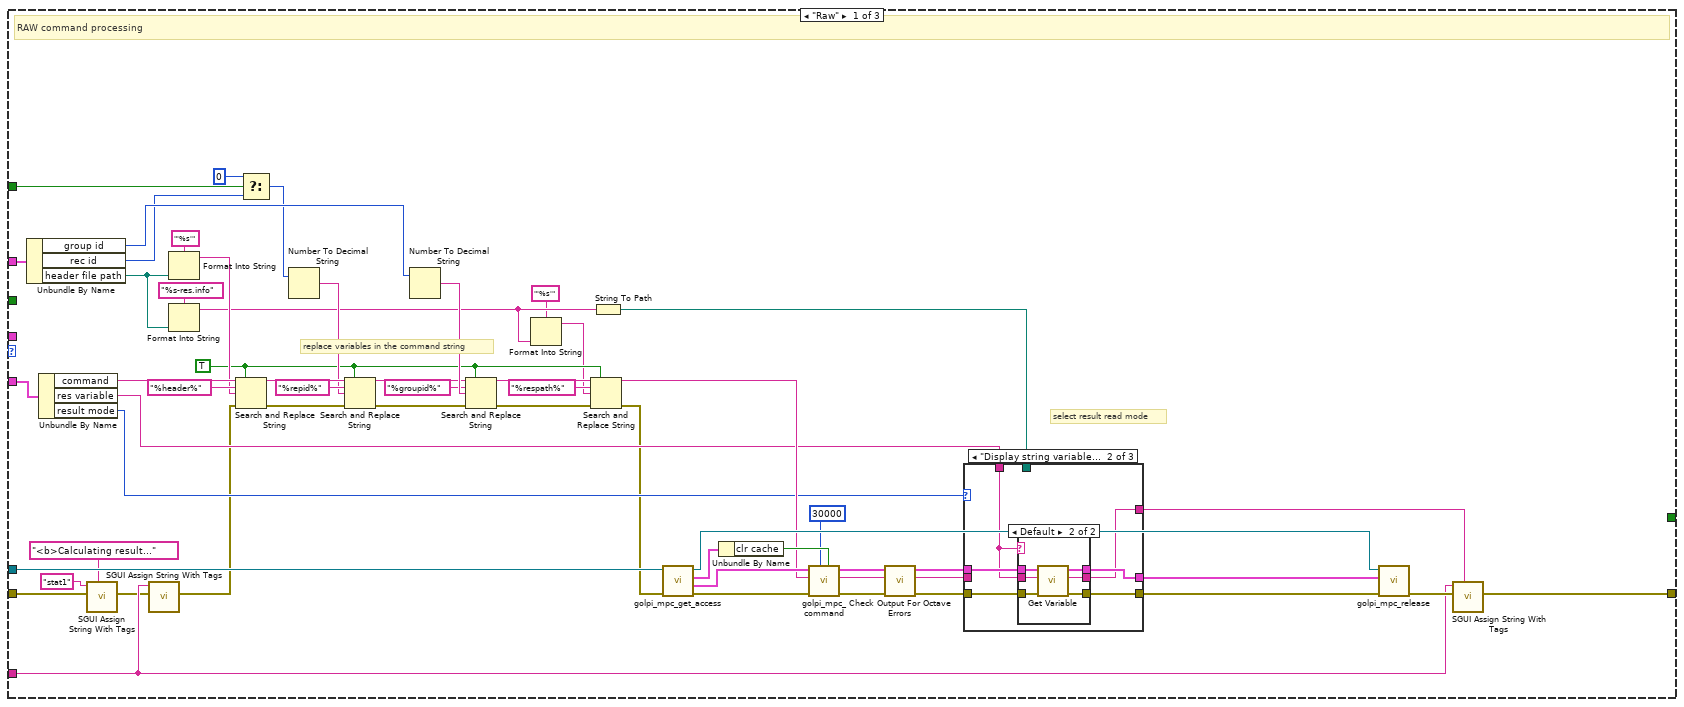
[diagram p3: hidden frame]
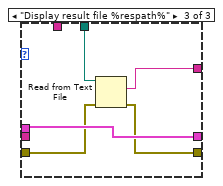
[diagram p6: hidden frame]
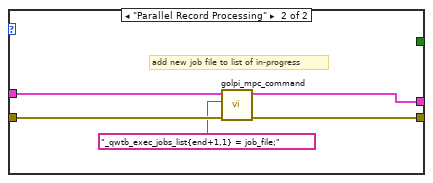
[diagram p7: hidden frame]
diagram:
  n1 = Unbundle By Name("session") -> ("processing setup.QWTB.unc once?"=w5:bool, "processing setup.QWTB"=w7:T101, "processing setup.mode"=w14:T98, "processing setup.calculate?"=w12:bool, "processing setup.raw mode"=w15:T99, "golpi"=w18:T96, "processing setup.call after avgs?"=w8:bool)
  n2 = Unbundle By Name("sequence item") -> ("group done?"=w9:bool, "rec id"=w3:i32)
  n3 = Greater?(x=w3, y=1) -> (0:w6:bool)
  n4 = Compound Arithmetic op=OR(invert w8, w9) -> (w11:bool)
  n5 = Compound Arithmetic op=AND(w6, w5) -> (w4:bool)
  n6 = Compound Arithmetic op=AND(w12, w11) -> (w13:bool)
  n7 = case shown="True" w13 {
    tunnel: "error in" -> [w21 w29]
    tunnel: w18 -> [_ w32]
    tunnel: [w21 w31] -> w17
    tunnel: "result string label" -> [_ w30]
    tunnel: w15 -> [_ w28]
    tunnel: "sequence item" -> [_ w27]
    tunnel: w14 -> [_ w26]
    tunnel: w8 -> [_ w25]
    tunnel: w7 -> [_ w24]
    tunnel: w4 -> [_ w23]
    tunnel: [_ w22] -> w1
    frame False {
    }
    frame True {
      # "execute Octave command"
      n8 = case shown="\"QWTB\"" w26 {
        tunnel: w32 -> [w86 w155 _]
        tunnel: [w80 w112 w189] -> w31
        tunnel: w30 -> [w77 w157 _]
        tunnel: w29 -> [w75 w159 w189]
        tunnel: w28 -> [w72 _ _]
        tunnel: w27 -> [w64 w167 _]
        tunnel: w25 -> [w42 _ _]
        tunnel: w24 -> [_ w154 _]
        tunnel: w23 -> [_ w142 _]
        tunnel: [_ w110 _] -> w22
        frame "Raw" {
          w53 = TRUE ("replace all? (F)")
          # "select result read mode"
          # "replace variables in the command string"
          # "RAW command processing"
          n9 = Unbundle By Name(w64) -> ("group id"=w57:i32, "rec id"=w41:i32, "header file path"=w67:path)
          n10 = Unbundle By Name(w72) -> ("command"=w71:string, "res variable"=w48:string, "result mode"=w47:T100)
          n11 = call-poly "SGUI Assign String With Tags.vi"("error in"=w75, "label(s) (empty)"="stat1", "string (empty)"="<b>Calculating result...") -> ("error out"=w76:errorcluster)  [unwired: 7 in, 1 out]
          n12 = call-poly "SGUI Assign String With Tags.vi"("error in"=w76, "label(s) (empty)"=w77) -> ("error out"=w43:errorcluster)  [unwired: 8 in, 1 out]
          n13 = Format Into String(format string="'%s'", w67) -> (resulting string=w63:string)  [unwired: 2 in, 1 out]
          n14 = Format Into String(format string="%s-res.info", w67) -> (resulting string=w37:string)  [unwired: 2 in, 1 out]
          n15 = Search and Replace String(replace all?=w53, input string=w71, search string="%header%", replace string=w63, error in=w43) -> (result string=w70:string, error out=w68:errorcluster)  [unwired: 3 in, 2 out]
          n16 = Select(t=0, s=w42, f=w41) -> (s? t:f=w40:i32)
          n17 = Number To Decimal String(number=w40) -> (decimal integer string=w62:string)  [unwired: 1 in]
          n18 = Search and Replace String(replace all?=w53, input string=w70, search string="%repid%", replace string=w62, error in=w68) -> (result string=w58:string, error out=w59:errorcluster)  [unwired: 3 in, 2 out]
          n19 = Number To Decimal String(number=w57) -> (decimal integer string=w61:string)  [unwired: 1 in]
          n20 = Search and Replace String(replace all?=w53, input string=w58, search string="%groupid%", replace string=w61, error in=w59) -> (result string=w54:string, error out=w55:errorcluster)  [unwired: 3 in, 2 out]
          n21 = Format Into String(format string="'%s'", w37) -> (resulting string=w38:string)  [unwired: 2 in, 1 out]
          n22 = Search and Replace String(replace all?=w53, input string=w54, search string="%respath%", replace string=w38, error in=w55) -> (result string=w52:string, error out=w44:errorcluster)  [unwired: 3 in, 2 out]
          n23 = String To Path(string=w37) -> (path=w46:path)
          n24 = call "golpi_mpc_get_access.vi"("error in"=w44, "golpi session ref"=w86) -> ("error out"=w87:errorcluster, "GOLPI ref out"=w85:T110, "golpi session out"=w84:T112, "golpi session ref out (copy)"=w82:T96)  [unwired: 4 in, 2 out]
          n25 = Unbundle By Name(w84) -> ("clr cache"=w83:bool)
          n26 = call "golpi_mpc_command.vi"("clear function cache before command? (False)"=w83, "timeout [ms]"=u32 30000, "error in"=w87, "command"=w52, "GOLPI ref in"=w85) -> ("error out"=w35:errorcluster, "read buffer"=w34:string, "GOLPI ref. out"=w51:T110)  [unwired: 4 in]
          n27 = call "Check Output For Octave Errors.vi"("error in"=w35, "read buffer"=w34) -> ("error out"=w33:errorcluster)  [unwired: 9 in]
          n28 = case shown="\"Display string variable\"" w47 {
            tunnel: w33 -> [w88 w96 w108]
            tunnel: w51 -> [w89 w95 w109]
            tunnel: [w88 w94 w107] -> w50
            tunnel: [w89 w93 w109] -> w49
            tunnel: w48 -> [_ w91 _]
            tunnel: [w90 w92 w105] -> w45
            tunnel: w34 -> [w90 _ _]
            tunnel: w46 -> [_ _ w106]
            frame "Display console output (only Octave)", Default {
            }
            frame "Display string variable" {
              n29 = case shown="Default" w91 {
                tunnel: w96 -> [w98 w104]
                tunnel: w95 -> [w97 w103]
                tunnel: [w98 w102] -> w94
                tunnel: [w97 w101] -> w93
                tunnel: w91 -> [_ w100]
                tunnel: [_ w99] -> w92
                frame "" {
                }
                frame Default {
                  n30 = call-poly "Get Variable.vi"("error in"=w104, "variable name"=w100, "GOLPI ref. in"=w103) -> ("error out"=w102:errorcluster, "value"=w99:string, "GOLPI ref. out"=w101:T110)  [unwired: 6 in]
                }
              }
            }
            frame "Display result file %respath%" {
              n31 = Read from Text File(file (use dialog)=w106, error in=w108) -> (text=w105:string, error out=w107:errorcluster)  [unwired: 2 in, 2 out]
            }
          }
          n32 = call "golpi_mpc_release.vi"("error in"=w50, "golpi ref or golpi session in"=w49, "golpi session ref"=w82) -> ("error out"=w81:errorcluster)  [unwired: 7 in, 1 out]
          n33 = call-poly "SGUI Assign String With Tags.vi"("error in"=w81, "label(s) (empty)"=w77, "string (empty)"=w45) -> ("error out"=w80:errorcluster)  [unwired: 7 in, 1 out]
        }
        frame "QWTB" {
          # "make parallel execution setup"
          # "execute directly or just add create job file"
          # "inhibit unc. multicore\nwhen parallel exec"
          # "force no uncertainty\nif not first reading and\nunc. calc. just once selected"
          # "QWTB command processing"
          n34 = Unbundle By Name(w154) -> ("qwtb timeout"=w152:i32, "multicore"=w149:T103, "exec mode"=w117:T105)
          n35 = Seconds To Date/Time(time stamp (now)="group time stamp") -> (date time rec=w126:T113)  [unwired: 1 in]
          n36 = call-poly "SGUI Assign String With Tags.vi"("error in"=w159, "label(s) (empty)"="stat1", "string (empty)"="<b>Calculating result...") -> ("error out"=w162:errorcluster)  [unwired: 7 in, 1 out]
          n37 = Unbundle By Name(w126) -> ("year"=w124:i32, "month"=w123:i32, "day of month"=w122:i32, "hour"=w121:i32, "minute"=w120:i32, "second"=w119:i32)
          n38 = Unbundle By Name(w167) -> ("header file path"=w156:path, "rec id"=w144:i32, "group id"=w153:i32)
          n39 = Equal?(x=w117, y=Meas_Proc_QWTB_Exec_Mode."Parallel Record Processing") -> (x = y?=w130:bool)
          n40 = Unbundle By Name(w149) -> ("jobs folder"=w125:path, "cores"=w148:i32, "mode"=w133:T1)
          n41 = call-poly "SGUI Assign String With Tags.vi"("error in"=w162, "label(s) (empty)"=w157) -> ("error out"=w158:errorcluster)  [unwired: 8 in, 1 out]
          n42 = Select(t=Meas_Proc_QWTB_Multicore_Type."Singlecore", s=w130, f=w133) -> (s? t:f=w132:T1)
          n43 = Format Into String(format string="pcfg = struct('mc_tmpdir','%s', 'time',struct('year',%d,'month',%d,'day',%d,'hour',%d,'minute',%d,'second',%d));\\n", w125, w124, w123, w122, w121, w120, w119) -> (resulting string=w118:string)  [unwired: 2 in, 1 out]
          n44 = property on="mode" class="Enum (strict)"() -> ("Strings []"=w146:string[])  [unwired: 2 in, 2 out]
          n45 = case shown="\"Multistation\"" w132 {
            tunnel: [w187 0 ("cores")] -> w147
            tunnel: w148 -> [w187 _]
            frame Default {
            }
            frame "Multistation" {
              # "start no servers"
            }
          }
          n46 = Index Array(array=w146, index=w132) -> (element=w145:string)
          n47 = call "golpi_mpc_get_access.vi"("error in"=w158, "golpi session ref"=w155) -> ("error out"=w165:errorcluster, "GOLPI ref out"=w171:T110, "golpi session out"=w170:T112, "golpi session ref out (copy)"=w168:T96)  [unwired: 4 in, 2 out]
          n48 = Select(t="none", s=w142, f="") -> (s? t:f=w143:string)
          n49 = Select(t="[job_file] = qwtb_exec_makejob", s=w130, f="qwtb_exec_algorithm") -> (s? t:f=w131:string)
          n50 = Multiply(x=w152, y=1000) -> (x*y=w150:i32)
          n51 = Unbundle By Name(w170) -> ("clr cache"=w169:bool)
          n52 = Format Into String(format string="cfg = struct('mc_method','%s', 'mc_procno',%d, 'mc_tmpdir','%s', 'parallel_cfg',pcfg);\n%s('%s', '%s', 1, %d, %d, 1, cfg);", initial string=w118, error in=w165, w145, w147, w125, w131, w156, w143, w144, w153) -> (resulting string=w164:string, error out=w166:errorcluster)
          n53 = call "golpi_mpc_command.vi"("clear function cache before command? (False)"=w169, "timeout [ms]"=w150, "error in"=w166, "command"=w164, "GOLPI ref in"=w171) -> ("error out"=w137:errorcluster, "read buffer"=w136:string, "GOLPI ref. out"=w115:T110)  [unwired: 4 in]
          n54 = call "Check Output For Octave Errors.vi"("error in"=w137, "read buffer"=w136) -> ("error out"=w139:errorcluster)  [unwired: 9 in]
          n55 = Compound Arithmetic op=AND(w139, invert w137) -> (w138:bool)
          n56 = case shown="True" w138 {
            tunnel: w137 -> [w181 w186]
            tunnel: w136 -> [_ w185]
            tunnel: [w181 w182] -> w116
            frame False {
            }
            frame True {
              # "QWTB error detected\n###note: workaround for GOLPI unable to detect multi-line errors"
              n57 = call <vilib>:"Error Cluster From Error Code.vi"("show call chain? (False)"=TRUE, "error in (no error)"=w186, "error message (\"\")"=w185, "error code (0)"=5000) -> ("error out"=w182:errorcluster)  [unwired: 5 in]
            }
          }
          n58 = case shown="\"Single-core\", Default" w117 {
            tunnel: w116 -> [w175 w180]
            tunnel: w115 -> [w173 w178]
            tunnel: [w173 w177] -> w114
            tunnel: [w174 w176] -> w113
            tunnel: [w172 _] -> w110
            frame "Single-core", Default {
              w172 = TRUE ("new result? (False)")
              n59 = call "Meas Proc QWTB Notify Result Queue.vi"("error in"=w175, "new result? (False)"=w172) -> ("error out"=w174:errorcluster)  [unwired: 8 in, 1 out]
            }
            frame "Parallel Record Processing" {
              # "add new job file to list of in-progress"
              n60 = call "golpi_mpc_command.vi"("error in"=w180, "command"="_qwtb_exec_jobs_list{end+1,1} = job_file;" ("format string"), "GOLPI ref in"=w178) -> ("error out"=w176:errorcluster, "GOLPI ref. out"=w177:T110)  [unwired: 6 in, 1 out]
            }
          }
          n61 = call "golpi_mpc_release.vi"("error in"=w113, "golpi ref or golpi session in"=w114, "golpi session ref"=w168) -> ("error out"=w112:errorcluster)  [unwired: 7 in, 1 out]
        }
        frame Default {
        }
      }
    }
  }
  "error out" <- w17
  "new result?" <- w1
